vi "Payload_Define.vi"(7 "Hex(T)":bool, 10 "Payload":u8[](array[numeric])=[0, 0, 0, 1, 2, 0, 28, 0] format="%.0x", 11 "Bytes":u32[](array[numeric])=[0, 4, 6]) -> (2 "Payload String":string, 3 "Read payload":u8[](array[numeric]) format="%.0x")   [LabVIEW 2024, in "Test_2.lvlib"]
uses:
  Test_2.lvlib
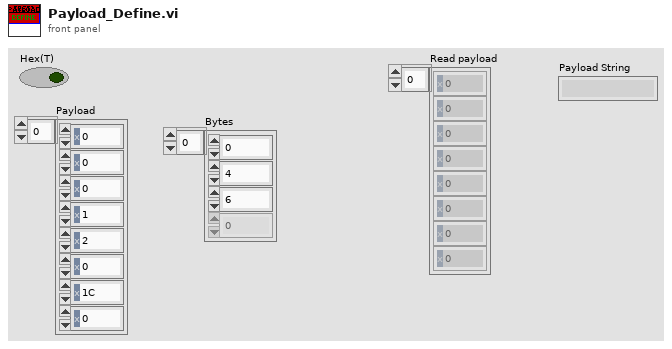
[diagram p1: front panel]
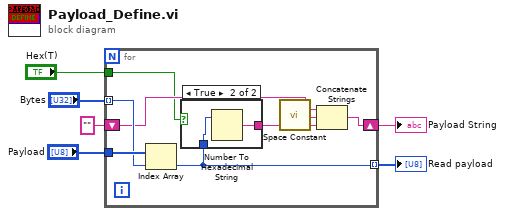
[diagram p0: block diagram]
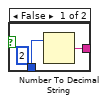
[diagram p2: hidden frame]
diagram:
  n1 = for {
    tunnel: "Bytes" -> [w13] mode=indexing
    tunnel: "Payload" -> [w14]
    tunnel: [w12] -> w4 mode=indexing
    shift-right: [w10] -> w1
    shift-left: "" -> [w9]
    tunnel: "Hex(T)" -> [w7]
    n2 = Index Array(array=w14, index=w13) -> (element=w12:u8)
    n3 = case shown="True" w7 {
      tunnel: w12 -> [w16 w17]
      tunnel: [w15 w18] -> w8
      frame False {
        (unwired) i16 2 ("width (-)")
        n4 = Number To Decimal String(number=w16) -> (decimal integer string=w15:string)  [unwired: 1 in]
      }
      frame True {
        n5 = Number To Hexadecimal String(2:w17) -> (0:w18:string)  [unwired: 1 in]
      }
    }
    n6 = call <vilib>:"Space Constant.vi"() -> ("String"=w11:string)
    n7 = Concatenate Strings(w9, w11, w8) -> (w10:string)
  }
  "Read payload" <- w4
  "Payload String" <- w1
